vi "Register.vi"(1 "TimeoutName":string, 2 "TimeoutInterface":refnum<class "ITimerTimeout.lvclass">, 3 "TimeoutTime(s)":dbl, 5 "error in (no error)":errorcluster) -> (15 "TimeoutID":u32, 19 "error out":errorcluster)   [LabVIEW 2020, in "LcTimer.lvclass"]
uses:
  LcTimer.lvclass
  ITimerTimeout_Interface/ITimerTimeout.lvclass
  private/TimeoutTask.vi
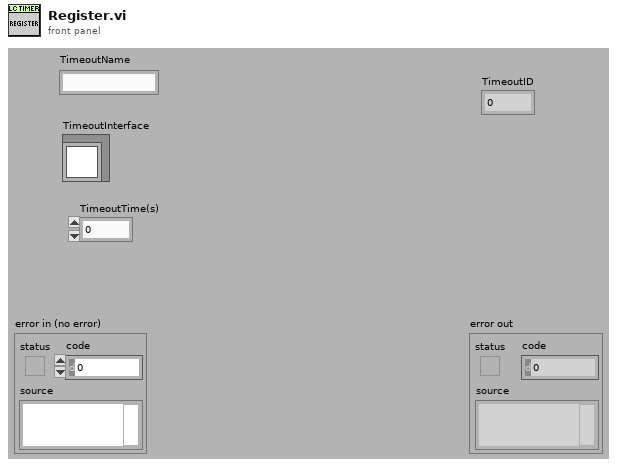
[diagram p1: front panel]
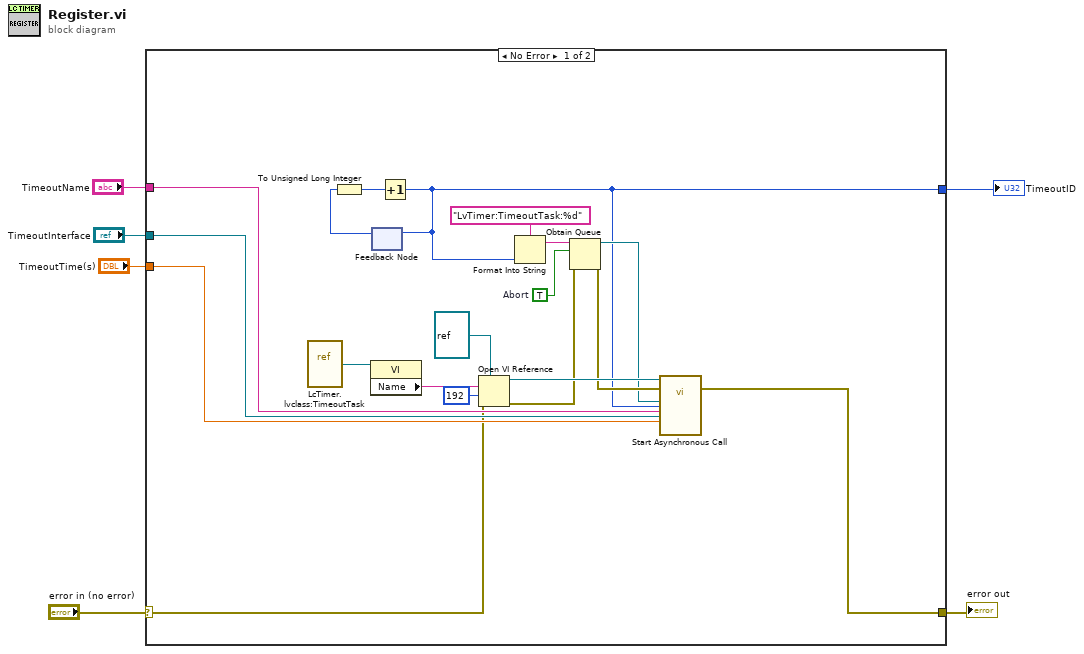
[diagram p0: block diagram]
diagram:
  n1 = case shown="No Error" "error in (no error)" {
    selector: "error in (no error)" -> [w7 w26]
    tunnel: [w8 w26] -> w5
    tunnel: [w12 _] -> w4
    tunnel: "TimeoutName" -> [w11 _]
    tunnel: "TimeoutInterface" -> [w10 _]
    tunnel: "TimeoutTime(s)" -> [w9 _]
    frame No Error {
      w21 = TRUE  # Abort
      n2 = vi-ref "LcTimer.lvclass:TimeoutTask.vi"() -> (w20:refnum<vi>)
      n3 = property class="VI"(reference=w20) -> ("Name"=w19:string)  [unwired: 1 in, 2 out]
      n4 = feedback #1() -> (w25:u32)  [unwired: 1 in]
      n5 = To Unsigned Long Integer(number=w25) -> (unsigned 32bit integer=w24:u32)
      n6 = Increment(x=w24) -> (x+1=w12:u32)
      n7 = feedback-in #1(w12) -> ()
      n8 = Open VI Reference(type specifier VI Refnum (for type only)=refnum<vi> refnum, vi path=w19, options=192, error in (no error)=w7) -> (vi reference=w16:refnum<vi>, error out=w15:errorcluster)  [unwired: 2 in]
      n9 = Format Into String(format string="LvTimer:TimeoutTask:%d", w12) -> (resulting string=w22:string)  [unwired: 2 in, 1 out]
      n10 = Obtain Queue(name (unnamed)=w22, element data type=w21, error in (no error)=w15) -> (queue out=w13:refnum<queue>, error out=w14:errorcluster)  [unwired: 2 in, 1 out]
      n11 = call-by-ref "Start Asynchronous Call"(reference=w16, error in=w14, "AbortQueue"=w13, "TimeoutID"=w12, "TimeoutName"=w11, "TimeoutInterface"=w10, "TimeoutTime(s)"=w9) -> (error out=w8:errorcluster)  [unwired: 14 in, 2 out]
    }
    frame Error {
    }
  }
  "error out" <- w5
  "TimeoutID" <- w4
